vi "Scroll_Pump_Error_Message.vi"(6 "Scroll Pump Message":string, 9 "Fault register":bool[](array[boolean]), 11 "Warning register":bool[](array[boolean])) -> ()   [LabVIEW 2014]
panel:
  in  "Exit":bool
  # "Fault due to excessive link voltage"
  # "Pump-controller temperature is below the minimum measurable value"
  # "Fault due to excessive motor current"
  # "Fault due to excessive pump-controller temperature"
  # "Pump-controller temperature sensor failure"
  # "Power stage failure"
  # "Output current is being restricted due to high pump-controller temperature"
  # "Hardware fault latch active"
  # "Fault due to a critical EEPROM problem (e.g. Parameter upload incomplete)"
  # "Pump-controller temperature is above the maximum measurable value"
  # "Parameter set upload required"
  # "Self test fault (e.g. Invalid software code)"
  # "Fault because the serial enable input went inactive whilst operating with a serial start command"
  # "Fault because the output frequency fell below the threshold for more than the allowable time (with an active start command)"
  # "Fault because the output frequency did not reach the threshold in the allowable time (following a start command)"
  # "Non-critical problem with EEPROM or other internal function"
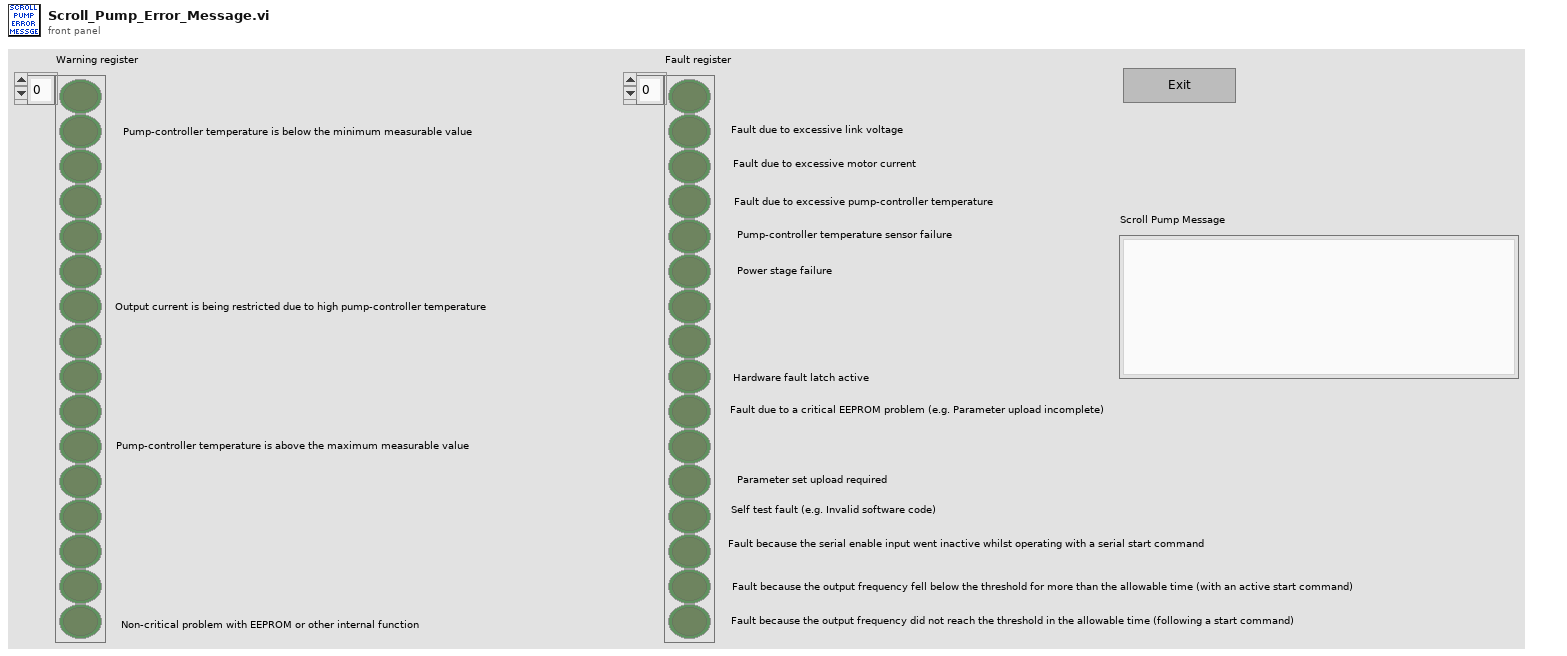
[diagram p1: front panel]
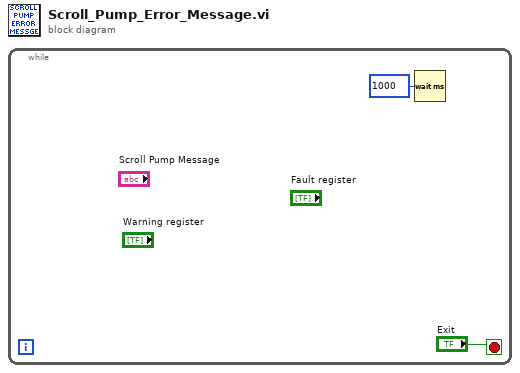
[diagram p0: block diagram]
diagram:
  n1 = while {
    stop <- "Exit" stop-if-true
    n2 = Wait (ms)(milliseconds to wait=u32 1000) -> ()  [unwired: 1 out]
  }
